vi "Add cell to table.vi"(0 "PdfP Table":refnum<k24>, 1 "Row Borders":T5={"Row"={"#"=0, "to #"=0}, "Cell Cluster"={"Font Ref"=refnum, "Leading"=18.0, "Horizontal Aligment"=enum."JUSTIFY", "Vertical Alignment"=enum."BOTTOM"}, "PdfPCell [ ]"=[]}, 2 "Image to Add [ ]":T6, 3 "Back Ground Color":u32(colorbox)=16777215, 5 "String":string, 7 "i":i32, 9 "Column Width (points)":dbl, 11 "error in (no error)":errorcluster) -> (4 "PdfP Table duplicate":refnum<k24>, 15 "error out":errorcluster)   [LabVIEW 2013]
doc: "Version 1.0\nDeveloped by Jean-Marc Simard\nCopyright © 2010, Exaprom Inc.\nAll rights reserved.\nLicense: BSD\n\nWith iTextSharp 4.1.6 (http://itextsharp.sourceforge.net)\nunder Mozilla Public License Version 1.1\n(http://www.mozilla.org/MPL/MPL-1.1.html)"
uses:
  C:/Users/MaxCorp/Documents/GitHub/TopView/DLL/itextsharp.dll
  DLL/itextsharp.dll
  Controls/Image to Add refnum [ ].ctl
  Controls/Cell Cluster.ctl
  Controls/Font size.ctl
  Controls/Texte alignement.ctl
  Controls/Cell Vertical alignment.ctl
  <vilib>/regexp/Match Regular Expression.xnode
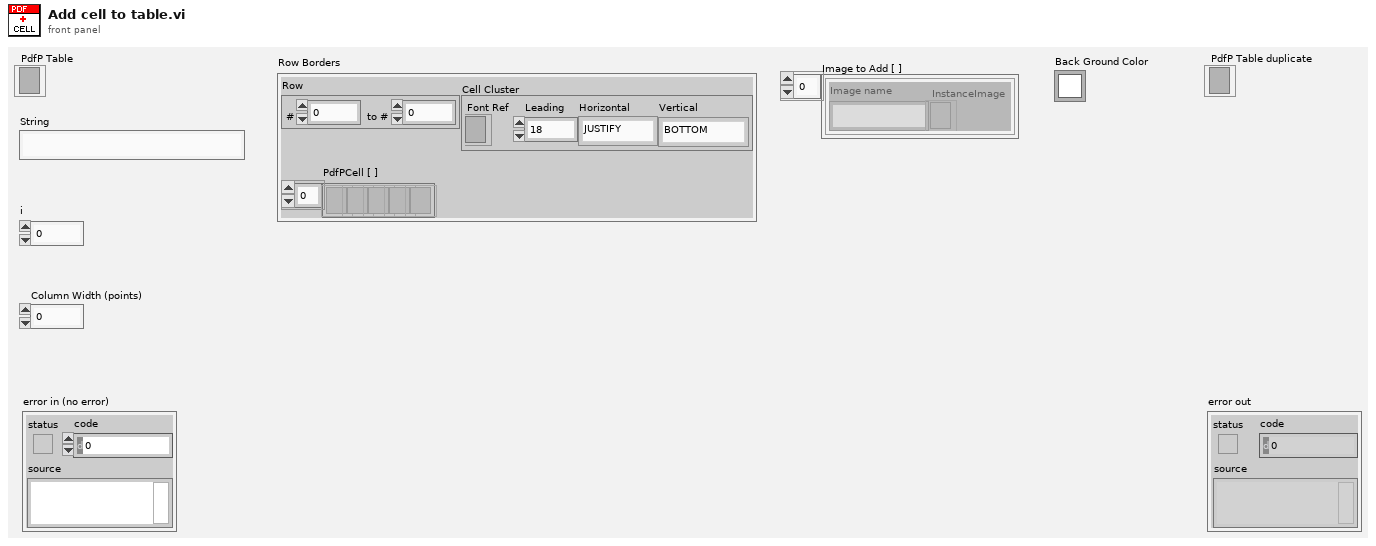
[diagram p1: front panel]
types:
  T1 = typedef "Cell Cluster.ctl" = cluster{"Font Ref":refnum<k24>, "Leading":T2, "Horizontal Aligment":T3, "Vertical Alignment":T4}
  T2 = typedef "Font size.ctl" = sgl
  T3 = typedef "Texte alignement.ctl" = enum16{"Select", "CENTER", "JUSTIFY", "LEFT", "RIGHT"}
  T4 = typedef "Cell Vertical alignment.ctl" = enum16{"TOP", "MIDDLE", "BOTTOM"}
  T5 = cluster{"Row":cluster{"#":i16, "to #":i16}, "Cell Cluster":T1, "PdfPCell [ ]":refnum<k24>[]}
  T6 = typedef "Image to Add refnum [ ].ctl" = cluster{"Image name":string, "InstanceImage":refnum<k24>}[]
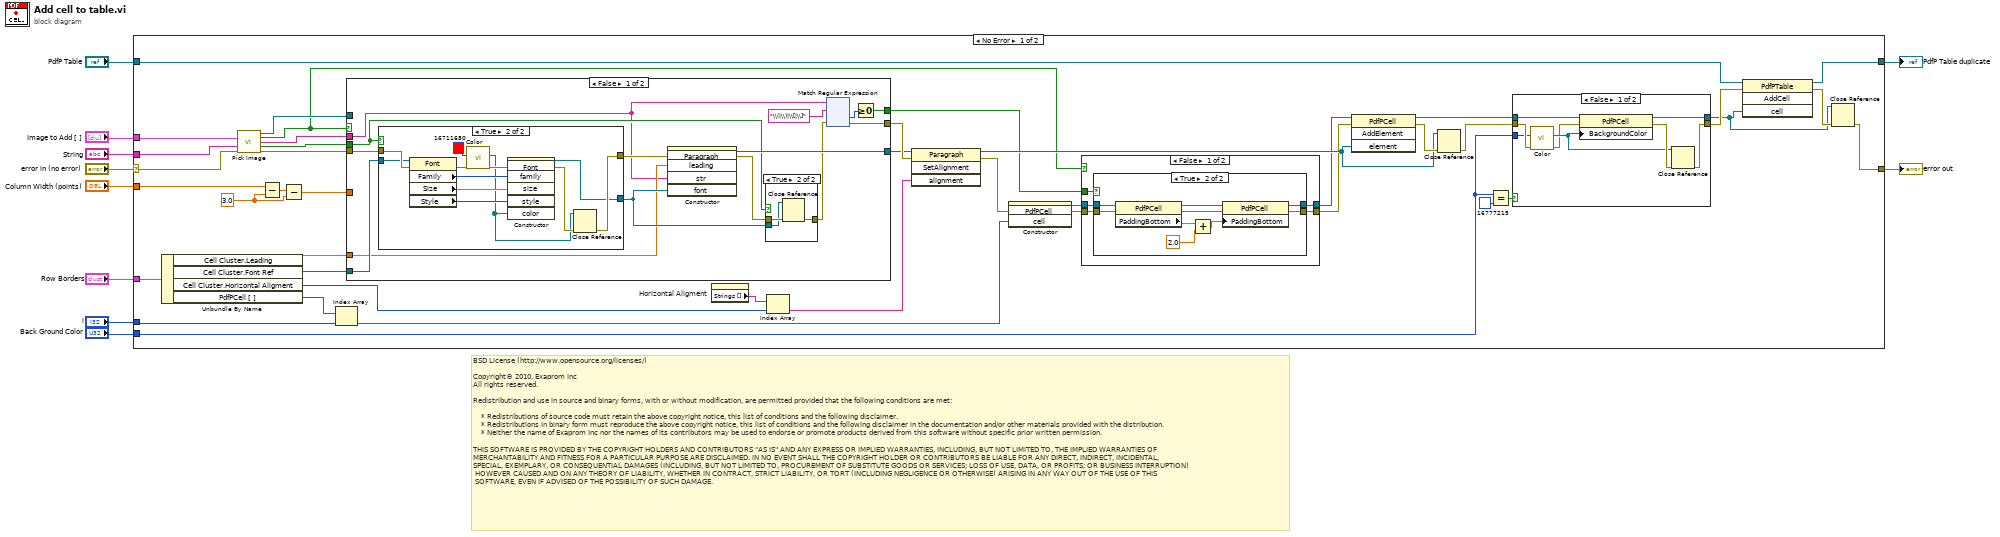
[diagram p0: block diagram]
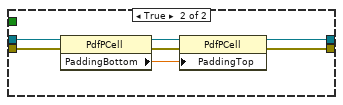
[diagram p3: hidden frame]
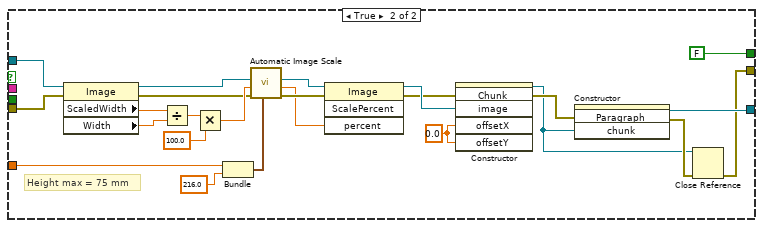
[diagram p7: hidden frame]
diagram:
  # "BSD License (http://www.opensource.org/licenses/)\n\nCopyright© 2010, Exaprom Inc\nAll rights reserved.\n\nRedistribution and use in source and binary forms, with or without modification, are permitted provided that the following conditions are met:\n\n    * Redistributions of source code must retain the above copyright notice, this list of conditions and the following disclaimer.\n    * Redistributions in binary form must reproduce the above copyright notice, this list of conditions and the following disclaimer in the documentation and/or other materials provided with the distribution.\n    * Neither the name of Exaprom Inc nor the names of its contributors may be used to endorse or promote products derived from this software without specific prior written permission.\n\nTHIS SOFTWARE IS PROVIDED BY THE COPYRIGHT HOLDERS AND CONTRIBUTORS \"AS IS\" AND ANY EXPRESS OR IMPLIED WARRANTIES, INCLUDING, BUT NOT LIMITED TO, THE IMPLIED WARRANTIES OF \nMERCHANTABILITY AND FITNESS FOR A PARTICULAR PURPOSE ARE DISCLAIMED. IN NO EVENT SHALL THE COPYRIGHT HOLDER OR CONTRIBUTORS BE LIABLE FOR ANY DIRECT, INDIRECT, INCIDENTAL,\nSPECIAL, EXEMPLARY, OR CONSEQUENTIAL DAMAGES (INCLUDING, BUT NOT LIMITED TO, PROCUREMENT OF SUBSTITUTE GOODS OR SERVICES; LOSS OF USE, DATA, OR PROFITS; OR BUSINESS INTERRUPTION)\n HOWEVER CAUSED AND ON ANY THEORY OF LIABILITY, WHETHER IN CONTRACT, STRICT LIABILITY, OR TORT (INCLUDING NEGLIGENCE OR OTHERWISE) ARISING IN ANY WAY OUT OF THE USE OF THIS\n SOFTWARE, EVEN IF ADVISED OF THE POSSIBILITY OF SUCH DAMAGE."
  n1 = case shown="No Error" "error in (no error)" {
    selector: "error in (no error)" -> [w25 w257]
    tunnel: [w29 w257] -> w9
    tunnel: [w52 w256] -> w8
    tunnel: "PdfP Table" -> [w12 w256]
    tunnel: "String" -> [w26 _]
    tunnel: "Image to Add [ ]" -> [w27 _]
    tunnel: "Column Width (points)" -> [w51 _]
    tunnel: "i" -> [w31 _]
    tunnel: "Back Ground Color" -> [w11 _]
    tunnel: "Row Borders" -> [w36 _]
    frame No Error {
      w49 = sgl 3.0 ("t")
      n2 = Unbundle By Name(w36) -> ("Cell Cluster.Leading"=w35:T2, "Cell Cluster.Font Ref"=w34:refnum<k24>, "Cell Cluster.Horizontal Aligment"=w33:T3, "PdfPCell [ ]"=w32:refnum<k24>[])
      n3 = call "Pick Image.vi"("Image to Add [ ]"=w27, "String"=w26, "error in (no error)"=w25) -> ("InstanceImage"=w23:refnum<k24>, "Valid Image?"=w14:bool, "String OUT"=w22:string, "Change Font Color?"=w21:bool, "error out"=w24:errorcluster)  [unwired: 8 out]
      n4 = Subtract(x=w51, y=w49) -> (x-y=w50:dbl)
      n5 = Subtract(x=w50, y=w49) -> (x-y=w48:dbl)
      n6 = Index Array(array=w32, index=w31) -> (element=w19:refnum<k24>)
      n7 = case shown="False" w14 {
        tunnel: w24 -> [w94 w240]
        tunnel: w34 -> [w99 _]
        tunnel: w35 -> [w92 _]
        tunnel: w23 -> [_ w255]
        tunnel: w48 -> [_ w253]
        tunnel: w21 -> [w93 _]
        tunnel: [w91 w233] -> w38
        tunnel: [w95 w237] -> w37
        tunnel: w22 -> [w89 _]
        tunnel: [w86 FALSE] -> w13
        frame False {
          n8 = case shown="True" w93 {
            tunnel: w94 -> [w218 w224]
            tunnel: w99 -> [w219 w223]
            tunnel: [w218 w222] -> w98
            tunnel: [w219 w221] -> w96
            frame False {
            }
            frame True {
              n9 = property class="Font"(reference=w223, error in=w224) -> (error out=w225:errorcluster, "Family"=w228:i32, "Size"=w229:sgl, "Style"=w230:i32)  [unwired: 1 out]
              n10 = call "Color.vi"("error in (no error)"=w225, "Color"=u32 16711680) -> ("error out"=w227:errorcluster, "Color"=w220:refnum<k24>)  [unwired: 8 out]
              n11 = constructor class="Font"(error in=w227, "family"=w228, "size"=w229, "style"=w230, "color"=w220) -> (reference out=w221:refnum<k24>, error out=w231:errorcluster)  [unwired: 2 in, 5 out]
              n12 = Close Reference(reference=w220, error in (no error)=w231) -> (error out=w222:errorcluster)
            }
          }
          n13 = constructor class="Paragraph"(error in=w98, "leading"=w92, "str"=w89, "font"=w96) -> (reference out=w95:refnum<k24>, error out=w97:errorcluster)  [unwired: 2 in, 4 out]
          n14 = case shown="True" w93 {
            tunnel: w97 -> [w214 w217]
            tunnel: [w214 w216] -> w90
            tunnel: w96 -> [_ w215]
            frame False {
            }
            frame True {
              n15 = Close Reference(reference=w215, error in (no error)=w217) -> (error out=w216:errorcluster)
            }
          }
          n16 = xnode "Match Regular Expression"("input string"=w89, "regular expression"="\\(|\\)|\\[|\\]", "error in"=w90) -> ("offset past match"=w87:i32, "error out"=w91:errorcluster)  [unwired: 1 in, 5 out]
          n17 = Greater Or Equal To 0?(x=w87) -> (x >= 0?=w86:bool)
        }
        frame True {
          w238 = sgl 0.0 ("offsetX")
          # "Height max = 75 mm"
          n18 = property class="Image"(reference=w255, error in=w240) -> (reference out=w254:refnum<k24>, error out=w239:errorcluster, "ScaledWidth"=w244:sgl, "Width"=w243:sgl)
          n19 = Divide(x=w244, y=w243) -> (x/y=w245:sgl)
          n20 = Multiply(x=w245, y=sgl 100.0) -> (x*y=w242:sgl)
          n21 = Bundle(w253, sgl 216.0) -> (w251:cluster{dbl, sgl})  [unwired: 1 out]
          n22 = call "Automatic Image Scale.vi"("Box"=w251, "error in (no error)"=w239, "Scale percent IN"=w242, "GetInstanceImage IN"=w254) -> ("error out"=w250:errorcluster, "Scale percent OUT"=w246:sgl, "GetInstanceImage OUT"=w249:refnum<k24>)  [unwired: 2 in, 3 out]
          n23 = invoke class="Image" method="ScalePercent"(reference=w249, error in=w250, "percent"=w246) -> (reference out=w248:refnum<k24>, error out=w247:errorcluster)  [unwired: 1 in, 2 out]
          n24 = constructor class="Chunk"(error in=w247, "image"=w248, "offsetX"=w238, "offsetY"=w238) -> (reference out=w234:refnum<k24>, error out=w236:errorcluster)  [unwired: 2 in, 4 out]
          n25 = constructor class="Paragraph"(error in=w236, "chunk"=w234) -> (reference out=w237:refnum<k24>, error out=w235:errorcluster)  [unwired: 2 in, 2 out]
          n26 = Close Reference(reference=w234, error in (no error)=w235) -> (error out=w233:errorcluster)
        }
      }
      n27 = property on="Horizontal Aligment" class="Enum (strict)"() -> ("Strings []"=w40:string[])  [unwired: 2 in, 2 out]
      n28 = Index Array(array=w40, index=w33) -> (element=w39:string)
      n29 = invoke class="Paragraph" method="SetAlignment"(reference=w37, error in=w38, "alignment"=w39) -> (reference out=w41:refnum<k24>, error out=w15:errorcluster)  [unwired: 1 in, 2 out]
      n30 = constructor class="PdfPCell"(error in=w15, "cell"=w19) -> (reference out=w18:refnum<k24>, error out=w16:errorcluster)  [unwired: 2 in, 2 out]
      n31 = case shown="False" w14 {
        tunnel: w16 -> [w54 w73]
        tunnel: [w53 w72] -> w20
        tunnel: w18 -> [w55 w71]
        tunnel: [w56 w69] -> w17
        tunnel: w13 -> [w57 _]
        frame False {
          n32 = case shown="True" w57 {
            tunnel: [w59 w66] -> w56
            tunnel: w55 -> [w59 w64]
            tunnel: w54 -> [w58 w63]
            tunnel: [w58 w65] -> w53
            frame False {
            }
            frame True {
              n33 = property class="PdfPCell"(reference=w64, error in=w63) -> (reference out=w67:refnum<k24>, error out=w68:errorcluster, "PaddingBottom"=w62:sgl)
              n34 = Add(x=w62, y=sgl 2.0) -> (x+y=w61:sgl)
              n35 = property class="PdfPCell"(reference=w67, error in=w68, "PaddingBottom"=w61) -> (reference out=w66:refnum<k24>, error out=w65:errorcluster)
            }
          }
        }
        frame True {
          n36 = property class="PdfPCell"(reference=w71, error in=w73) -> (reference out=w70:refnum<k24>, error out=w74:errorcluster, "PaddingBottom"=w75:sgl)
          n37 = property class="PdfPCell"(reference=w70, error in=w74, "PaddingTop"=w75) -> (reference out=w69:refnum<k24>, error out=w72:errorcluster)
        }
      }
      n38 = invoke class="PdfPCell" method="AddElement"(reference=w17, error in=w20, "element"=w41) -> (reference out=w43:refnum<k24>, error out=w44:errorcluster)  [unwired: 1 in, 2 out]
      n39 = Close Reference(reference=w41, error in (no error)=w44) -> (error out=w42:errorcluster)
      n40 = Equal?(x=w11, y=u32 16777215 ("Color")) -> (x = y?=w46:bool)
      n41 = case shown="False" w46 {
        tunnel: w43 -> [w83 w85]
        tunnel: w42 -> [w78 w84]
        tunnel: [w82 w85] -> w28
        tunnel: [w80 w84] -> w45
        tunnel: w11 -> [w77 _]
        frame False {
          n42 = call "Color.vi"("error in (no error)"=w78, "Color"=w77) -> ("error out"=w76:errorcluster, "Color"=w79:refnum<k24>)  [unwired: 8 out]
          n43 = property class="PdfPCell"(reference=w83, error in=w76, "BackgroundColor"=w79) -> (reference out=w82:refnum<k24>, error out=w81:errorcluster)
          n44 = Close Reference(reference=w79, error in (no error)=w81) -> (error out=w80:errorcluster)
        }
        frame True {
        }
      }
      n45 = invoke class="PdfPTable" method="AddCell"(reference=w12, error in=w45, "cell"=w28) -> (reference out=w52:refnum<k24>, error out=w30:errorcluster)  [unwired: 1 in, 2 out]
      n46 = Close Reference(reference=w28, error in (no error)=w30) -> (error out=w29:errorcluster)
    }
    frame Error {
    }
  }
  "error out" <- w9
  "PdfP Table duplicate" <- w8
